vi "Devolve_PDF_pela_TAG.vi"(6 "caminho_relacao_instrumento_PDF_txt":string="Certificados_calibracao\\relacao_instrumento_pdf.txt", 8 "TAG":string) -> (1 "found?":bool, 2 "path":path, 4 "TAG existe?":bool)   [LabVIEW 2019]
uses:
  <vilib>/Utility/config.llb/Read Key (String).vi
  <vilib>/Utility/config.llb/NI_LVConfig.lvlib
panel:
  # "essa VI abre o arquivo txt \"relacao_instrumento_pdf.txt\" que relaciona cada TAG com um determinado arquivo pdf que deverá ser seu certificado de calibração\no caminho_PDF contém o nome do arquivo txt e a pasta onde ele está, se a VI que chamou essa subVI estiver no PC SERVER, deve-se rodar localmente, \ncaso contrário, irá rodar pela REDE. Ao abrir o caminho path do arquivo txt, pela ATG recebida, é possível pegar a chave PDF que contém o caminho path do \narquivo PDF vinculado aquela TAG."
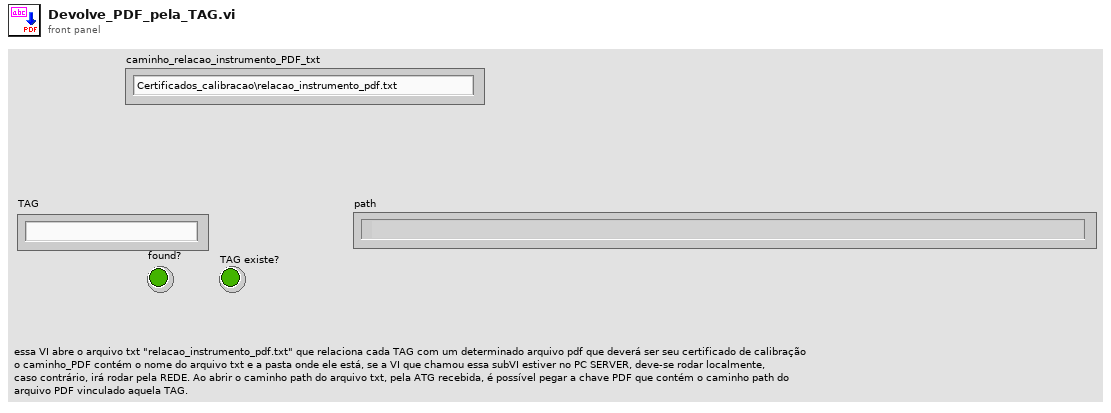
[diagram p1: front panel]
types:
  T1 = typedef "NI_LVConfig.lvlib/Config Data RefNum.ctl" = refnum<k1>
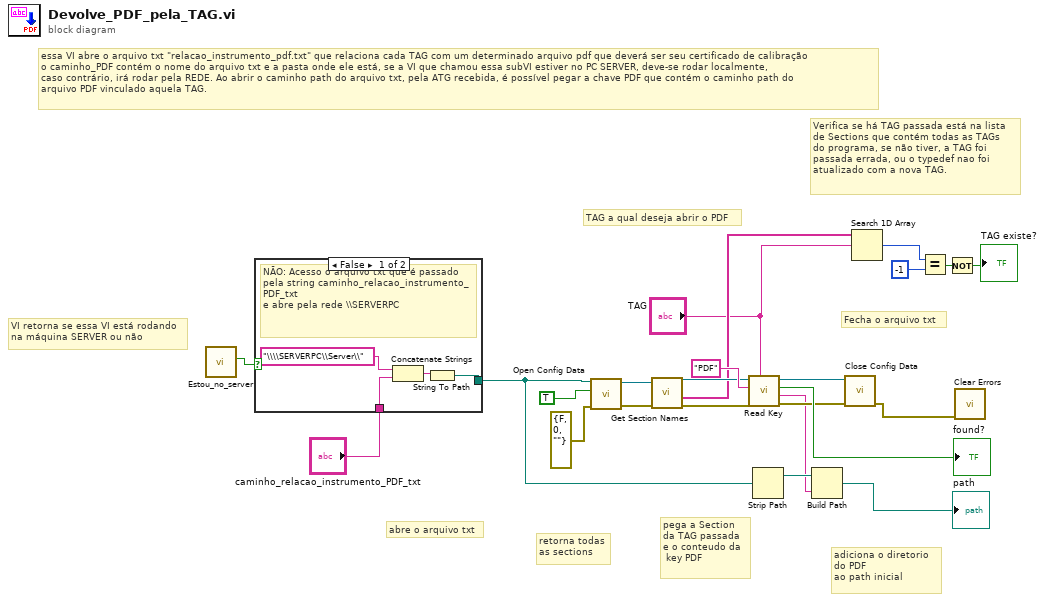
[diagram p0: block diagram]
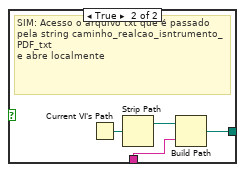
[diagram p2: hidden frame]
diagram:
  # "Fecha o arquivo txt"
  # "adiciona o diretorio \ndo PDF \nao path inicial"
  # "pega a Section \nda TAG passada\ne o conteudo da\n key PDF"
  # "retorna todas\nas sections"
  # "abre o arquivo txt"
  # "Verifica se há TAG passada está na lista \nde Sections que contém todas as TAGs\ndo programa, se não tiver, a TAG foi\npassada errada, ou o typedef nao foi \natualizado com a nova TAG."
  # "TAG a qual deseja abrir o PDF"
  # "VI retorna se essa VI está rodando\nna máquina SERVER ou não"
  # "essa VI abre o arquivo txt \"relacao_instrumento_pdf.txt\" que relaciona cada TAG com um determinado arquivo pdf que deverá ser seu certificado de calibração\no caminho_PDF contém o nome do arquivo txt e a pasta onde ele está, se a VI que chamou essa subVI estiver no PC SERVER, deve-se rodar localmente, \ncaso contrário, irá rodar pela REDE. Ao abrir o caminho path do arquivo txt, pela ATG recebida, é possível pegar a chave PDF que contém o caminho path do \narquivo PDF vinculado aquela TAG."
  n1 = call "Estou_no_server.vi"() -> ("Estou no serve?"=w6:bool)  [unwired: 11 in]
  n2 = case shown="False" w6 {
    tunnel: [w25 w30] -> w5
    tunnel: "caminho_relacao_instrumento_PDF_txt" -> [w26 w29]
    frame False {
      # "NÃO: Acesso o arquivo txt que é passado pela string caminho_relacao_instrumento_PDF_txt\ne abre pela rede \\\\SERVERPC"
      n3 = Concatenate Strings("\\\\SERVERPC\\Server\\", w26) -> (w24:string)
      n4 = String To Path(string=w24) -> (path=w25:path)
    }
    frame True {
      # "SIM: Acesso o arquivo txt que é passado pela string caminho_realcao_isntrumento_PDF_txt\ne abre localmente"
      n5 = Current VI's Path() -> (path=w28:path)
      n6 = Strip Path(path=w28) -> (stripped path=w31:path)  [unwired: 1 out]
      n7 = Build Path(base path=w31, name or relative path=w29) -> (appended path=w30:path)
    }
  }
  n8 = call <vilib>:"Open Config Data.vi"("error in (no error)"=errorcluster {"status"=FALSE, "code"=0, "source"=""}, "create file if necessary (T)"=TRUE, "configuration file path"=w5) -> ("error out"=w18:errorcluster, "refnum"=w19:T1)  [unwired: 6 in, 1 out]
  n9 = call <vilib>:"Get Section Names.vi"("error in (no error)"=w18, "refnum"=w19) -> ("error out"=w17:errorcluster, "section names"=w15:string[], "refnum out"=w16:T1)  [unwired: 7 in]
  n10 = call-poly <vilib>:"Read Key.vi"("section"="TAG", "error in (no error)"=w17, "key"="PDF", "refnum"=w16) -> ("error out"=w8:errorcluster, "value"=w3:string, "found?"=→"found?":bool, "refnum out"=w9:T1)  [unwired: 4 in]
  n11 = Strip Path(path=w5) -> (stripped path=w4:path)  [unwired: 1 out]
  n12 = Build Path(base path=w4, name or relative path=w3) -> (appended path=→"path":path)
  n13 = call <vilib>:"Close Config Data.vi"("error in (no error)"=w8, "refnum"=w9) -> ("error out"=w7:errorcluster)  [unwired: 8 in, 1 out]
  n14 = Search 1D Array(1D array=w15, element="TAG") -> (index of element=w13:i32)  [unwired: 1 in]
  n15 = Equal?(x=w13, y=-1) -> (x = y?=w11:bool)
  n16 = Not(x=w11) -> (.not. x?=→"TAG existe?":bool)
  n17 = call <vilib>:"Clear Errors.vi"("error in (no error)"=w7) -> ()  [unwired: 5 in, 2 out]
